vi "CleanUp.vi"(8 "ErrorIn":errorcluster caption="Error In", 11 "ObjectIn":refnum<class "testttt.lvclass"> caption="Object In") -> (0 "ErrorOut":errorcluster caption="Error Out", 3 "ObjectOut":refnum<class "testttt.lvclass"> caption="Object Out")   [LabVIEW 2018, in "testttt.lvclass"]
uses:
  testttt.lvclass
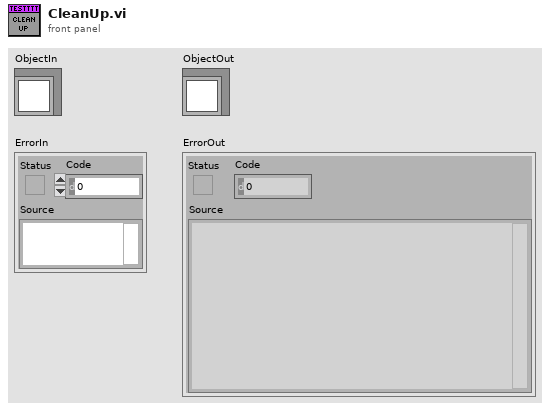
[diagram p1: front panel]
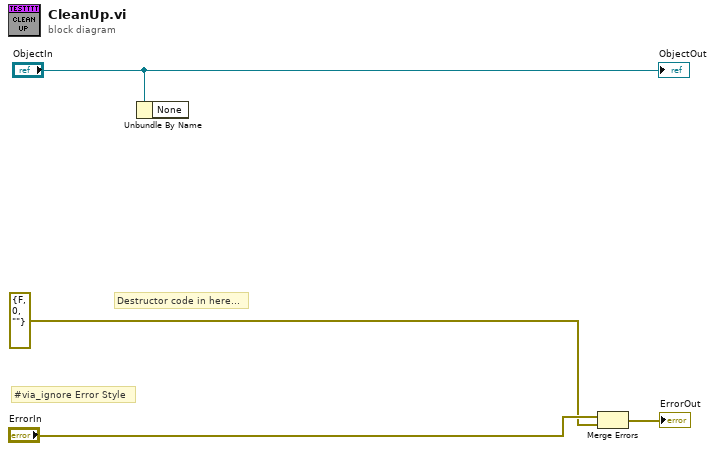
[diagram p0: block diagram]
diagram:
  # "#via_ignore Error Style"
  # "Destructor code in here..."
  n1 = Unbundle By Name("ObjectIn") -> ()  [unwired: 1 out]
  n2 = Merge Errors("ErrorIn", errorcluster {"status"=FALSE, "code"=0, "source"=""} ("error in (no error)")) -> (→"ErrorOut":errorcluster)
  "ObjectOut" <- "ObjectIn"
